vi "Recieve Set Output.vi"(6 "Output value":refnum<class "Mag Lab Result.lvclass">, 8 "error in (no error)":errorcluster, 9 "Requestor":string, 10 "Requestee":string, 11 "Mag Lab Hardware in":refnum<class "Mag Lab Hardware.lvclass">) -> (0 "error out":errorcluster, 3 "Mag Lab Hardware out":refnum<class "Mag Lab Hardware.lvclass">)   [LabVIEW 2015, in "Mag Lab Hardware.lvclass"]
uses:
  Mag Lab Hardware.lvclass
  Mag Lab Result/Mag Lab Result.lvclass
  Mag Lab Root/Mag Lab Root.lvclass/Mag Lab Root.ctl
  Mag Lab Result/Mag Lab Result.lvclass/Mag Lab Result.ctl
  <vilib>/ActorFramework/Actor/Actor.lvclass/Actor.ctl
  Mag Lab Root Messages/Recieve Response with Result Msg/Recieve Response with Result Msg.lvclass/Recieve Response with Result Msg.ctl
  <vilib>/ActorFramework/Message Enqueuer/Message Enqueuer.lvclass/Message Enqueuer.ctl
  <vilib>/ActorFramework/Message Enqueuer/Enqueue.vi
  <vilib>/ActorFramework/Message Priority Queue/Priority Enqueue.vi
  Mag Lab Root Messages/Recieve Response with Result Msg/Recieve Response with Result Msg.lvclass
  Mag Lab Root/Mag Lab Root.lvclass
  <vilib>/ActorFramework/Actor/Actor.lvclass
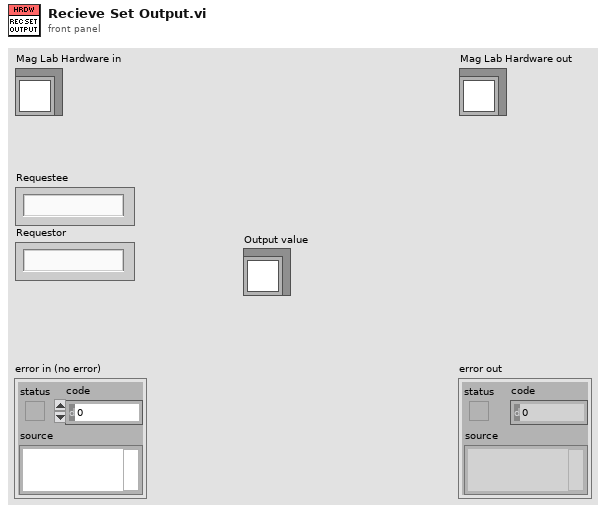
[diagram p1: front panel]
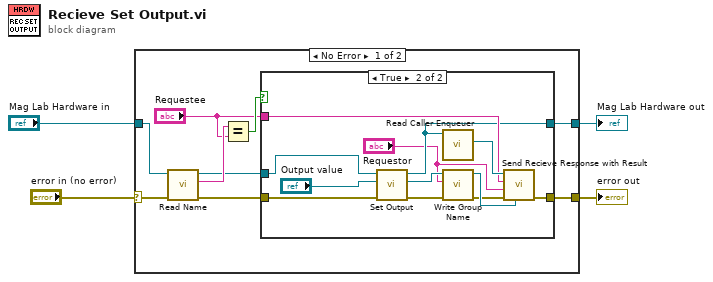
[diagram p0: block diagram]
diagram:
  n1 = case shown="No Error" "error in (no error)" {
    selector: "error in (no error)" -> [w10 w29]
    tunnel: [w13 w29] -> w1
    tunnel: [w12 w28] -> w2
    tunnel: "Mag Lab Hardware in" -> [w11 w28]
    frame No Error {
      n2 = call "Read Name.vi"("error in (no error)"=w10, "Mag Lab Root in"=w11) -> ("error out"=w6:errorcluster, "Name"=w9:string, "Mag Lab Root out"=w7:refnum<class "Mag Lab Hardware.lvclass">)  [unwired: 7 in]
      n3 = Equal?(x=w9, y="Requestee") -> (x = y?=w8:bool)
      n4 = case shown="True" w8 {
        tunnel: [w14 w24] -> w13
        tunnel: [w15 w23] -> w12
        tunnel: w7 -> [w15 w27]
        tunnel: "Requestee" -> [_ w25]
        tunnel: w6 -> [w14 w22]
        frame False {
        }
        frame True {
          n5 = call-dynamic "Set Output.vi"("error in (no error)"=w22, "Output value"="Output value", "Mag Lab Hardware in"=w27) -> ("error out"=w19:errorcluster, "Actual output value"=w21:refnum<class "Mag Lab Result.lvclass">, "Mag Lab Hardware out"=w23:refnum<class "Mag Lab Hardware.lvclass">)  [unwired: 6 in]
          n6 = call <vilib>:"Read Caller Enqueuer.vi"("Actor"=w23) -> ("Caller Enqueuer"=w26:refnum<class "Message Enqueuer.lvclass">)  [unwired: 10 in]
          n7 = call "Write Group Name.vi"("error in (no error)"=w19, "Group Name"="Requestor", "Mag Lab Result in"=w21) -> ("error out"=w18:errorcluster, "Mag Lab Result out"=w20:refnum<class "Mag Lab Result.lvclass">)  [unwired: 7 in]
          n8 = call "Send Recieve Response with Result.vi"("Result"=w20, "error in (no error)"=w18, "Requestor"="Requestor", "Requestee"=w25, "Message Enqueuer"=w26) -> ("error out"=w24:errorcluster)  [unwired: 5 in, 1 out]
        }
      }
    }
    frame Error {
    }
  }
  "error out" <- w1
  "Mag Lab Hardware out" <- w2
